vi "Save LVS.vi"(8 "error in (no error)":errorcluster, 10 "LVS Data":T4 {"Data OUT"."Parameter Time Series"."time offset" format="%.3f"; "Data OUT"."Parameter Time Series"."Gain" format="%.1f"; "Data OUT"."Parameter Time Series"."Offset" format="%.1f"; "Data OUT"."Parameter Time Series"."List 1" items=["Motor-Pos", "Motor-Vel", "Lx Position-in-Head", "Ly Position-in-Head", "Lz Position-in-Head", "Lx Velocity-in-Head", "Ly Velocity-in-Head", "Lz Velocity-in-Head", "Ll Velocity-in-Head", "Lr Velocity-in-Head", "Lx Accel-in-Head", "Ly Accel-in-Head", "Lz Accel-in-Head", "Rx Position-in-Head", "Ry Position-in-Head", "Rz Position-in-Head", "Rx Velocity-in-Head", "Ry Velocity-in-Head", "Rz Velocity-in-Head", "Rl Velocity-in-Head", "Rr Velocity-in-Head", "Rx Accel-in-Head", "Ry Accel-in-Head", "Rz Accel-in-Head", "Global Trigger", "", "", ""]; "Data OUT"."Parameter Impuls Series"."Gain" format="%.1f"; "Data OUT"."Parameter Impuls Series"."Offset" format="%.1f"}, 11 "Path (in)":path) -> (0 "error out":errorcluster, 3 "Path (out)":path)   [LabVIEW 2014]
uses:
  type-defs/TD_Statemachine-Data.ctl
  type-defs/TD_Time Series.ctl
  type-defs/TD_Impulse Parameter.ctl
  <userlib>/_OpenG.lib/file/file.llb/Convert File Extension (Path)__ogtk.vi
  core.lvlib
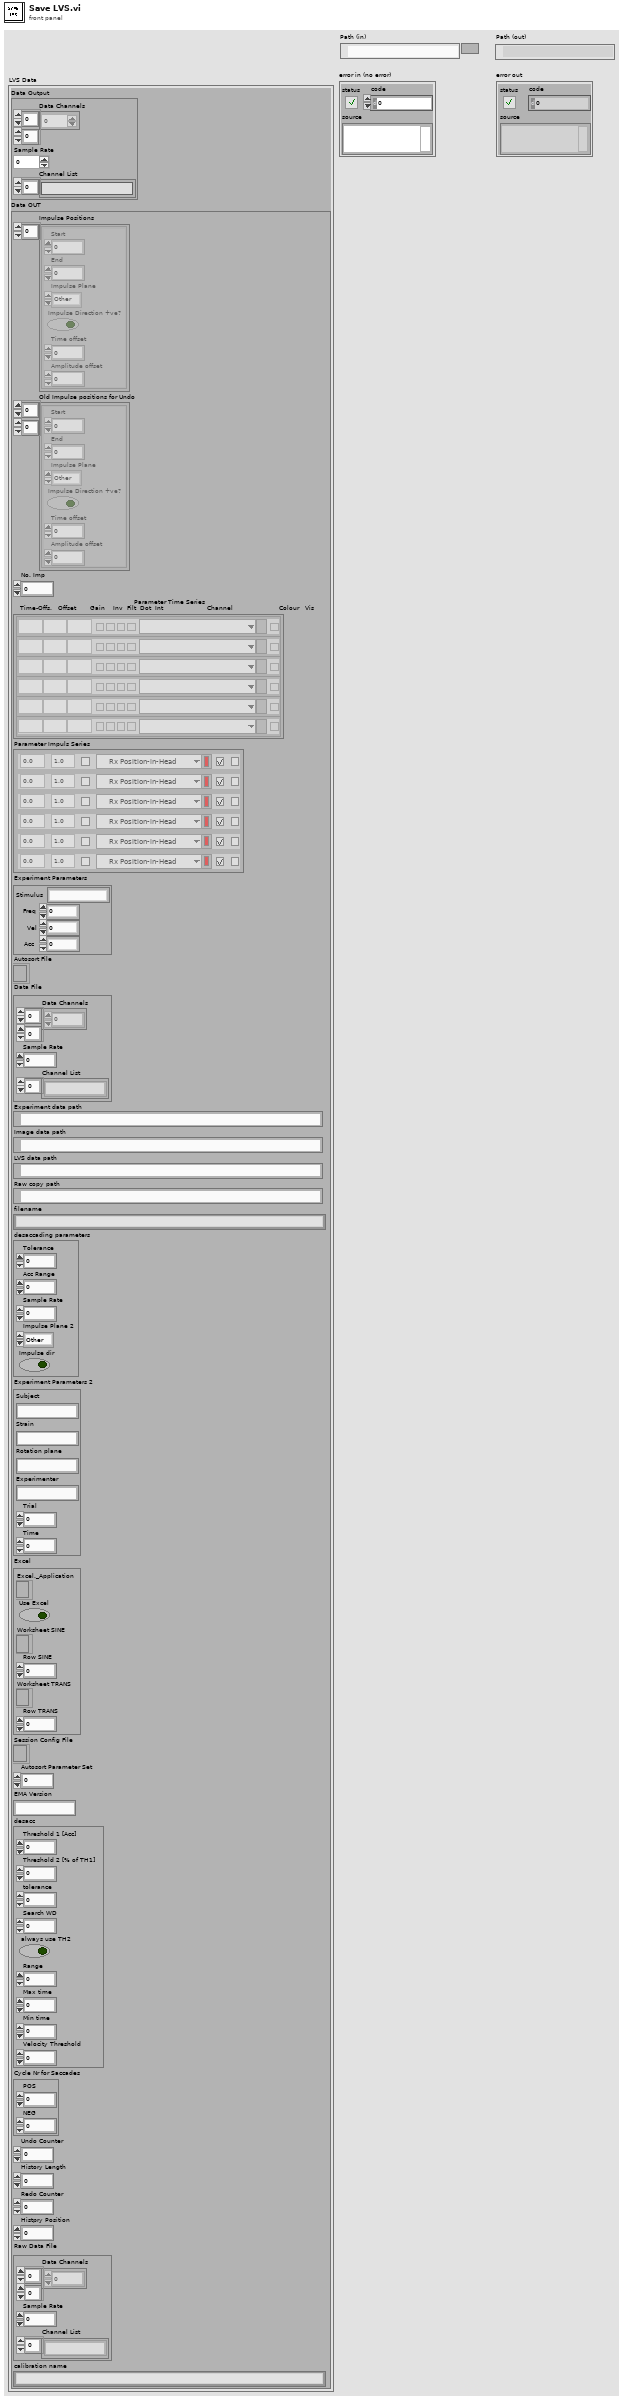
[diagram p1: front panel]
types:
  T1 = typedef "core.lvlib/TD_Statemachine-Data.ctl" = cluster{"Impulse Positions":cluster{"Start":i32, "End":i32, "Impulse Plane":enum16{"Other", "Yaw", "Pitch", "Roll", "LARP", "RALP"}, "Impulse Direction +ve?":bool, "Time offset":i32, "Amplitude offset":dbl}[], "Old Impulse positions for Undo":cluster{"Start":i32, "End":i32, "Impulse Plane":enum16{"Other", "Yaw", "Pitch", "Roll", "LARP", "RALP"}, "Impulse Direction +ve?":bool, "Time offset":i32, "Amplitude offset":dbl}[][], "No. Imp":i32, "Parameter Time Series":T2, "Parameter Impuls Series":T3, "Experiment Parameters":cluster{"Freq":dbl, "Vel":i32, "Acc":i32, "Stimulus":string}, "Autosort File":refnum<file>, "Data File":cluster{"Data Channels":dbl[][], "Sample Rate":i32, "Channel List":string[]}, "Experiment data path":path, "Image data path":path, "LVS data path":path, "Raw copy path":path, "filename":string, "desaccading parameters":cluster{"Tolerance":i32, "Acc Range":dbl, "Sample Rate":i32, "Impulse Plane 2":enum16{"Other", "Yaw", "Pitch", "Roll", "LARP", "RALP"}, "Impulse dir":bool}, "Experiment Parameters 2":cluster{"Subject":string, "Strain":string, "Rotation plane":string, "Experimenter":string, "Trial":dbl, "Time":dbl}, "Excel":cluster{"Excel._Application":refnum<k7>, "Use Excel":bool, "Worksheet SINE":refnum<k7>, "Row SINE":i32, "Worksheet TRANS":refnum<k7>, "Row TRANS":i32}, "Session Config File":refnum<file>, "Autosort Parameter Set":i32, "EMA Version":string, "desacc ":cluster{"Threshold 1 [Acc]":dbl, "Threshold 2 [% of TH1]":i32, "tolerance":i32, "Search WD ":dbl, " always use TH2":bool, "Range":dbl, "Max time":dbl, "Min time":dbl, "Velocity Threshold":i32}, "Cycle Nr for Saccades":cluster{"POS":i32, "NEG":i32}, "Undo Counter":i32, "History Length":i32, "Redo Counter":i32, "Histpry Position":i32, "Raw Data File":cluster{"Data Channels":dbl[][], "Sample Rate":i32, "Channel List":string[]}, "calibration name":string}
  T2 = typedef "core.lvlib/TD_Time Series.ctl" = cluster{"time offset":dbl, "Offset":dbl, "Gain":dbl, "inverse":bool, "filter data":bool, "dots":bool, "interpolate":bool, "List 1":u16, "Color Box":u32, "Boolean":bool}[]
  T3 = typedef "core.lvlib/TD_Impulse Parameter.ctl" = cluster{"Color":u32, "Visible":bool, "Channel":u16, "Invert":bool, "Desaccade":bool, "Offset":dbl, "Gain":dbl}[]
  T4 = cluster{"Data Output":cluster{"Data Channels":dbl[][], "Sample Rate":i32, "Channel List":string[]}, "Data OUT":T1}
  T5 = enum16{"open", "replace", "create", "open or create", "replace or create", "replace or create with confirmation"}
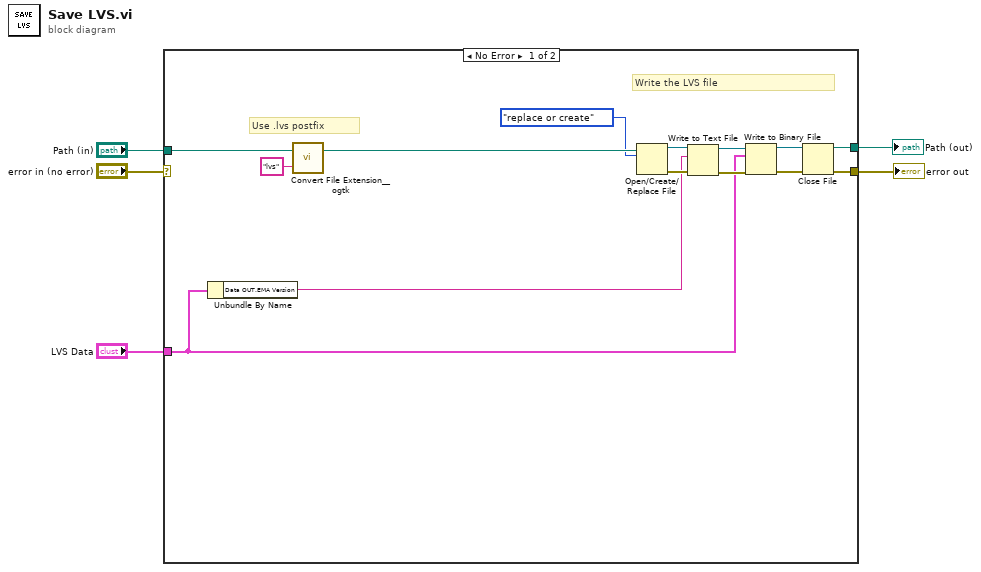
[diagram p0: block diagram]
diagram:
  n1 = case shown="No Error" "error in (no error)" {
    selector: "error in (no error)" -> [_ w21]
    tunnel: "Path (in)" -> [w19 w20]
    tunnel: "LVS Data" -> [w8 _]
    tunnel: [w16 w21] -> w2
    tunnel: [w15 w20] -> w1
    frame No Error {
      # "Write the LVS file"
      # "Use .lvs postfix"
      n2 = Unbundle By Name(w8) -> ("Data OUT.EMA Version"=w11:string)
      n3 = call-poly <userlib>:"Convert File Extension__ogtk.vi"("new ending (none)"="lvs", "file name"=w19) -> ("new filename"=w18:path)  [unwired: 1 out]
      n4 = Open/Create/Replace File(file path (use dialog)=w18, operation (0:open)=T5."replace or create") -> (refnum out=w12:refnum<file>, error out=w13:errorcluster)  [unwired: 4 in, 1 out]
      n5 = Write to Text File(file (use dialog)=w12, text=w11, error in=w13) -> (refnum out=w9:refnum<file>, error out=w10:errorcluster)  [unwired: 1 in, 1 out]
      n6 = Write to Binary File(file (use dialog)=w9, data=w8, error in=w10) -> (refnum out=w7:refnum<file>, error out=w6:errorcluster)  [unwired: 3 in, 1 out]
      n7 = Close File(refnum=w7, error in=w6) -> (path=w15:path, error out=w16:errorcluster)
    }
    frame Error {
    }
  }
  "error out" <- w2
  "Path (out)" <- w1
